vi "RUN 01 reset arms.vi"   [LabVIEW 2016]
types:
  T1 = typedef "LVHSConnector.ctl" = refnum<class "BrickReference.lvclass">
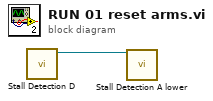
[diagram p0: block diagram]
diagram:
  n1 = call "Stall Detection D.vi"() -> ("NXT/EV3"=w1:T1)  [unwired: 11 in]
  n2 = call "Stall Detection A lower.vi"("NXT/EV3"=w1) -> ()  [unwired: 10 in, 1 out]
